vi "host.vi"() -> ()   [LabVIEW 2009]
uses:
  <vilib>/rvi/interface/nirviOpenFPGA/nirviOpenFPGA.xnode
  FPGA Bitfiles/spartan3E.lvproj_FPGA Target_LIA_FPGA.vi.lvbitx
  LIA_FPGA.vi
  <vilib>/FPGAPlugInAG/Spartan-3E Starter Board/nirviIntfOpen_Spartan-3E Starter Board.vi
  <vilib>/rvi/interface/nirviReadWriteControl/nirviReadWriteControl.xnode
  <vilib>/Utility/error.llb/Error Cluster From Error Code.vi
  <vilib>/rvi/errors/niLvFpgaAdjustHostInterfaceError.vi
  <vilib>/rvi/interface/common/niFpgaNodeNameForErrorReporting.ctl
  <vilib>/rvi/errors/niLvFpgaWhatHappensToTopLevelVI.ctl
  <vilib>/rvi/interface/nirviMethod/nirviMethod.xnode
  <vilib>/RVI Host/nirviSupport.llb/nirviErrorClusterFromErrorCode.vi
  <vilib>/rvi/errors/niLvFpgaReportInternalErrorWithAdditionalInfo.vi
  <vilib>/LabVIEW Targets/FPGA/XUPSpartan3E/Spartan3E_ReadBigControlVI.vi
  <vilib>/Utility/error.llb/Merge Errors.vi
  <vilib>/rvi/interface/nirviCloseFPGA/nirviCloseFPGA.xnode
  <vilib>/FPGAPlugInAG/Spartan-3E Starter Board/nirviIntfClose_Spartan-3E Starter Board.vi
  vi.lib/LabVIEW Targets/nilvcse/nilvcse.dll
panel:
  in  "Sampling Frequency":dbl=50000.0 min=1000.0 max=50000.0
  in  "stop":bool
  out "degree":dbl
  out "r":dbl
  out "y":dbl
  out "x":dbl
  out "f":dbl format="%.2g"
  in  "dec2":i16=1
  in  "nominal freq":dbl=1000.0 min=500.0 max=5000.0
  in  "dec1":i16=1000
  in  "stages":i8=1 min=1 max=2
  in  "decimation":i16=1000
  # "Sampling Frequency"
  # "CIC First Decimation"
  # "CIC Second Decimation"
  # "MA Stages"
  # "MA Decimation"
  # "PLL Nominal Frequency"
  # "PLL Frequency Output"
  # "LIA Output"
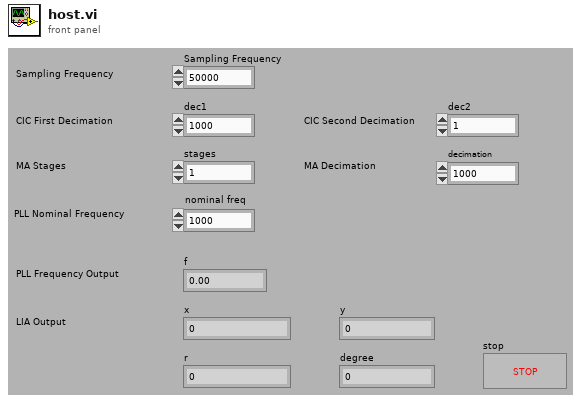
[diagram p1: front panel]
types:
  T1 = typedef "niFpgaNodeNameForErrorReporting.ctl" = enum16{"Open FPGA VI Reference", "Read/Write Control", "Invoke Method: Abort", "Invoke Method: Acknowledge IRQ", "Invoke Method: Download", "Invoke Method: FIFO.Configure", "Invoke Method: FIFO.Read", "Invoke Method: FIFO.Start", "Invoke Method: FIFO.Stop", "Invoke Method: FIFO.Write", "Invoke Method: Reset", "Invoke Method: Run", "Invoke Method: Wait on IRQ", "Close FPGA VI Reference"}
  T2 = typedef "niLvFpgaWhatHappensToTopLevelVI.ctl" = enum16{"top level VI scripted behind XNode", "top level VI inlined behind XNode"}
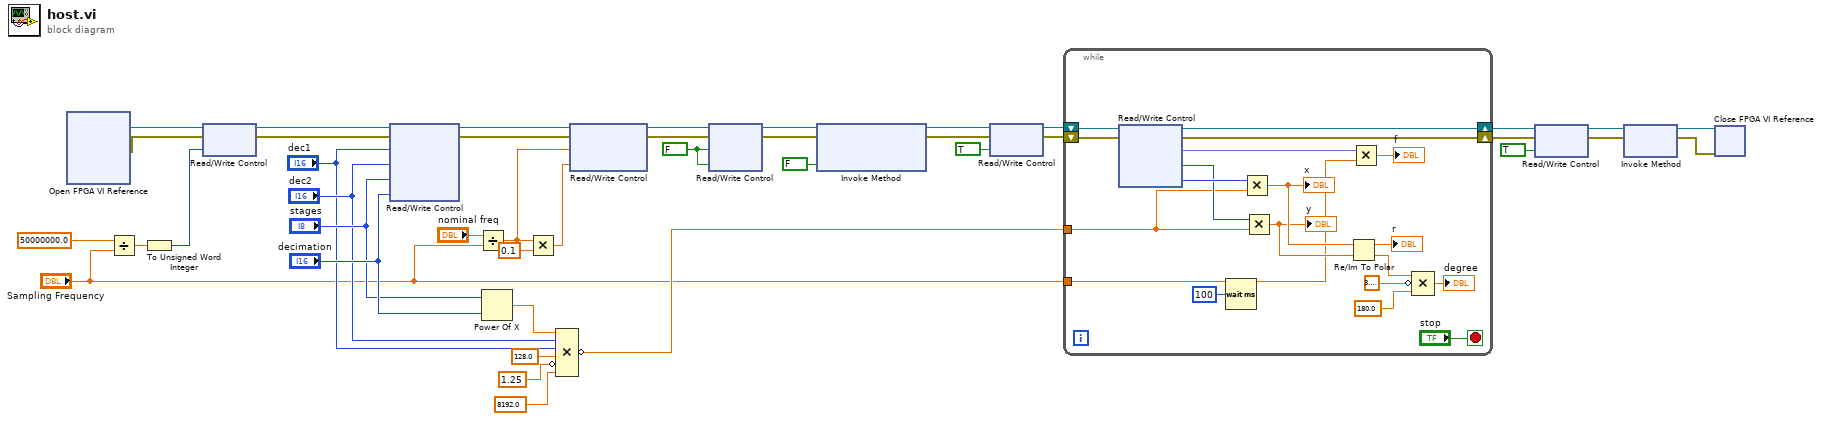
[diagram p0: block diagram]
diagram:
  w18 = FALSE ("start")
  n1 = xnode "Open FPGA VI Reference"() -> ("FPGA VI Reference Out"=w12:refnum<k20>, "error out"=w10:errorcluster)  [unwired: 1 in]
  n2 = Divide(x=50000000.0, y="Sampling Frequency") -> (x/y=w7:dbl)
  n3 = To Unsigned Word Integer(number=w7) -> (unsigned 16bit integer=w6:u16)
  n4 = xnode "Read/Write Control"("FPGA VI Reference In"=w12, "error in"=w10, "Period"=w6) -> ("FPGA VI Reference Out"=w11:refnum<k20>, "error out"=w9:errorcluster)
  n5 = xnode "Read/Write Control"("FPGA VI Reference In"=w11, "error in"=w9, "dec1"="dec1", "dec2"="dec2", "stages"="stages", "decimation"="decimation") -> ("FPGA VI Reference Out"=w41:refnum<k20>, "error out"=w40:errorcluster)
  n6 = Divide(x="nominal freq", y="Sampling Frequency") -> (x/y=w3:dbl)
  n7 = Power Of X(1:"decimation", 2:"stages") -> (0:w36:dbl)
  n8 = Multiply(x=w3, y=0.1) -> (x*y=w1:dbl)
  n9 = Compound Arithmetic op=MULTIPLY(w36, "dec2", "dec1", 128.0, invert 1.25, 8192.0 ("value")) -> (invert w31:dbl)
  n10 = xnode "Read/Write Control"("FPGA VI Reference In"=w41, "error in"=w40, "nominal freq"=w3, "K"=w1) -> ("FPGA VI Reference Out"=w22:refnum<k20>, "error out"=w21:errorcluster)
  n11 = xnode "Read/Write Control"("FPGA VI Reference In"=w22, "error in"=w21, "start"=w18, "stop"=w18) -> ("FPGA VI Reference Out"=w20:refnum<k20>, "error out"=w19:errorcluster)
  n12 = xnode "Invoke Method"("FPGA VI Reference In"=w20, "error in"=w19, "Wait Until Done (F)"=FALSE) -> ("FPGA VI Reference Out"=w27:refnum<k20>, "error out"=w25:errorcluster)
  n13 = xnode "Read/Write Control"("FPGA VI Reference In"=w27, "error in"=w25, "start"=TRUE) -> ("FPGA VI Reference Out"=w26:refnum<k20>, "error out"=w24:errorcluster)
  n14 = while {
    shift-right: [w55] -> w30
    shift-left: w26 -> [w60]
    shift-right: [w54] -> w29
    shift-left: w24 -> [w59]
    tunnel: w31 -> [w56]
    tunnel: "Sampling Frequency" -> [w43]
    stop <- "stop" stop-if-true
    n15 = xnode "Read/Write Control"("FPGA VI Reference In"=w60, "error in"=w59) -> ("FPGA VI Reference Out"=w55:refnum<k20>, "error out"=w54:errorcluster, "f"=w44:fxp<+/-,32,0>, "channelQ"=w57:i64, "channelI"=w58:i64)
    n16 = Wait (ms)(milliseconds to wait=u32 100) -> ()  [unwired: 1 out]
    n17 = Multiply(x=w58, y=w56) -> (x*y=w53:dbl)
    "x" <- w53
    n18 = Multiply(x=w57, y=w56) -> (x*y=w52:dbl)
    "y" <- w52
    n19 = Re/Im To Polar(2:w52, 3:w53) -> (0:w50:dbl, 1:→"r":dbl)
    n20 = Multiply(x=w44, y=w43) -> (x*y=→"f":dbl)
    n21 = Compound Arithmetic op=MULTIPLY(w50, invert 3.141592653589793, 180.0 ("value")) -> (→"degree":dbl)
  }
  n22 = xnode "Read/Write Control"("FPGA VI Reference In"=w30, "error in"=w29, "stop"=TRUE) -> ("FPGA VI Reference Out"=w16:refnum<k20>, "error out"=w15:errorcluster)
  n23 = xnode "Invoke Method"("FPGA VI Reference In"=w16, "error in"=w15) -> ("FPGA VI Reference Out"=w14:refnum<k20>, "error out"=w13:errorcluster)
  n24 = xnode "Close FPGA VI Reference"("FPGA VI Reference In"=w14, "error in"=w13) -> ()  [unwired: 1 out]
